vi "K to C Demo.vi"   [LabVIEW 2012, in "Temp Converter.lvlib"]
uses:
  Temp Converter.lvlib
  K to C (1D dbl).vi
  K to C (2D dbl).vi
  K to C (dbl).vi
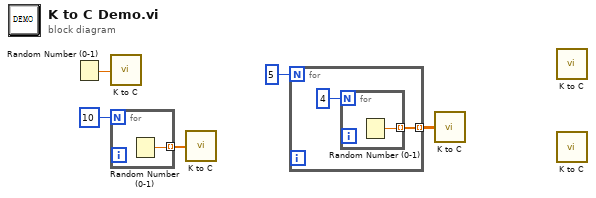
[diagram p0: block diagram]
diagram:
  n1 = Random Number (0-1)() -> (number: 0 to 1=w5:dbl)
  n2 = call-poly "K to C.vi"("K"=w5) -> ()  [unwired: 1 out]
  n3 = for {
    N: 10 -> [_]
    tunnel: [w6] -> w3 mode=indexing
    n4 = Random Number (0-1)() -> (number: 0 to 1=w6:dbl)
  }
  n5 = call-poly "K to C.vi"("K"=w3) -> ()  [unwired: 1 out]
  n6 = for {
    N: 5 -> [_]
    tunnel: [w7] -> w1 mode=indexing
    n7 = for {
      N: 4 -> [_]
      tunnel: [w9] -> w7 mode=indexing
      n8 = Random Number (0-1)() -> (number: 0 to 1=w9:dbl)
    }
  }
  n9 = call-poly "K to C.vi"("K"=w1) -> ()  [unwired: 1 out]
  n10 = call-poly "K to C.vi"() -> ()  [unwired: 1 in, 1 out]
  n11 = call-poly "K to C.vi"() -> ()  [unwired: 1 in, 1 out]
